vi "channel and task settings.vi"(8 "Error In":errorcluster, 10 "Channel and Task settings":T1={"All Channels to read"=[], "Task names"=[], "number of samples \nper channel [k]"=0.0, "sampling rate [kHz]"=1.0}, 11 "mode (R)":T2=enum."read") -> (0 "Error out":errorcluster, 2 "Channel and Task settings":T1={"All Channels to read"=[], "Task names"=[], "number of samples \nper channel [k]"=0.0, "sampling rate [kHz]"=1.0})   [LabVIEW 2011]
doc: "Functional Global Variable for the algorithm settings. The used method as well as the max. Iteration steps and the tolerance can be given. In addition, the algorithm can be told to use boundaries (if possible)."
uses:
  controls/FGV_Action.ctl
  controls/Channel and Task settings.ctl
panel:
  # "Input"
  # "Output"
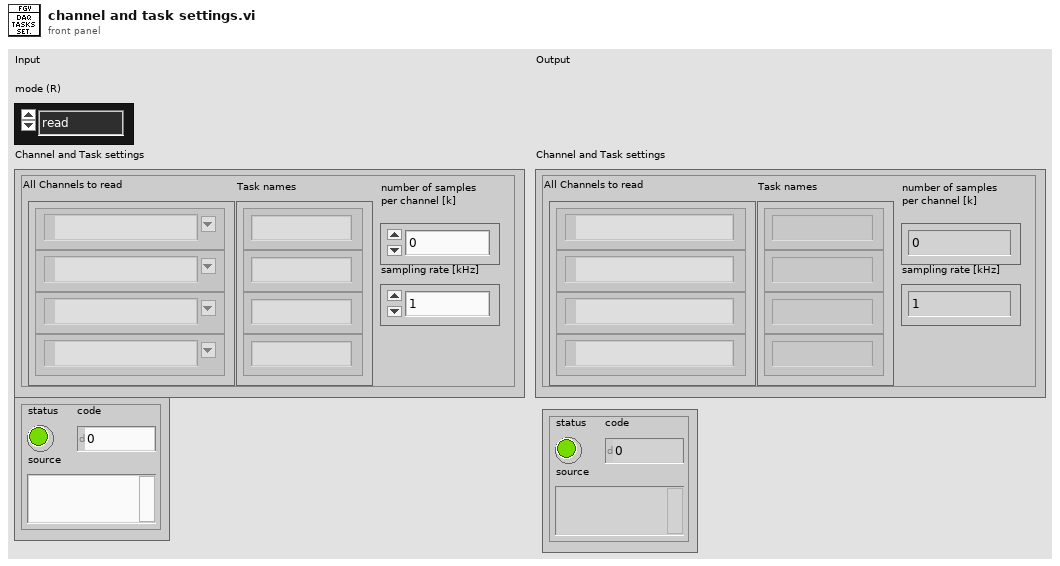
[diagram p1: front panel]
types:
  T1 = typedef "Channel and Task settings.ctl" = cluster{"All Channels to read":tag[], "Task names":string[], "number of samples \nper channel [k]":dbl, "sampling rate [kHz]":dbl}
  T2 = typedef "FGV_Action.ctl" = enum16{"set to default", "read", "write"}
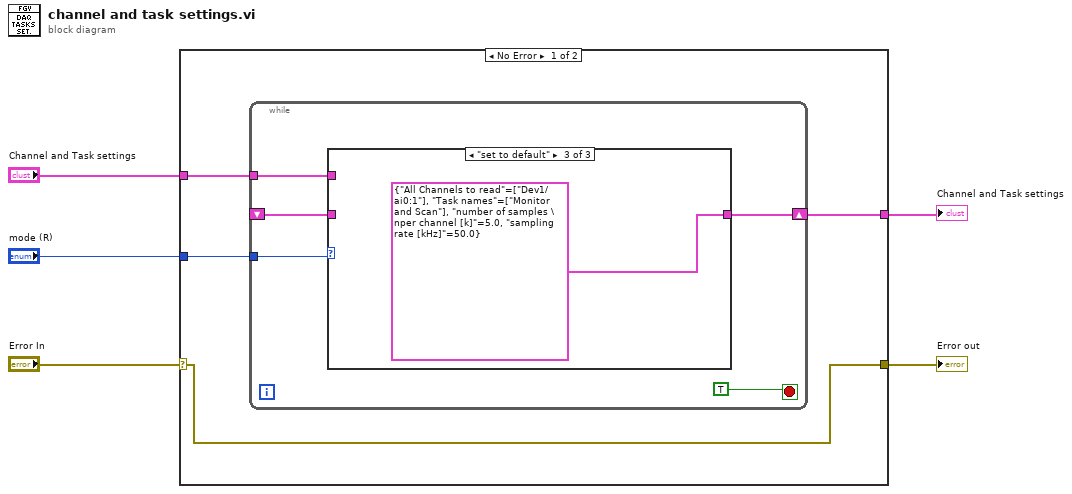
[diagram p0: block diagram]
diagram:
  n1 = case shown="No Error" "Error In" {
    selector: "Error In" -> [w6 w19]
    tunnel: "mode (R)" -> [w9 _]
    tunnel: [w6 w19] -> w3
    tunnel: "Channel and Task settings" -> [w8 w18]
    tunnel: [w7 w18] -> w1
    frame No Error {
      n2 = while {
        tunnel: w9 -> [w13]
        tunnel: w8 -> [w12]
        shift-right: [w10] -> w7
        shift-left: _ -> [w11]
        stop <- TRUE stop-if-true
        n3 = case shown="\"set to default\"" w13 {
          tunnel: w12 -> [_ w16 _]
          tunnel: w11 -> [w15 _ _]
          tunnel: [w15 w16 T1 {"All Channels to read"=["Dev1/ai0:1"], "Task names"=["Monitor and Scan"], "number of samples \nper channel [k]"=5.0, "sampling rate [kHz]"=50.0} ("Channel and Task settings")] -> w10
          frame "read", Default {
          }
          frame "write" {
          }
          frame "set to default" {
          }
        }
      }
    }
    frame Error {
    }
  }
  "Error out" <- w3
  "Channel and Task settings" <- w1
